vi "array_to_table.vi"() -> ()   [LabVIEW 2022 SP3]
panel:
  out "Table":string[][](table)
  in  "?":dbl[][](array[numeric])
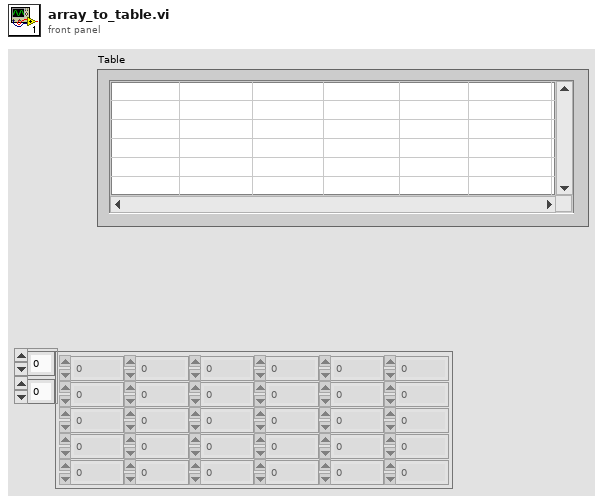
[diagram p1: front panel]
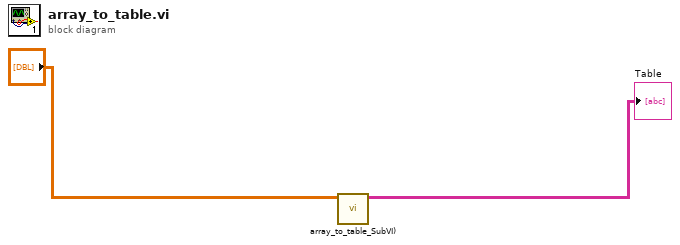
[diagram p0: block diagram]
diagram:
  n1 = call "array_to_table_SubVI).vi"("Array in"="?") -> ("Array out"=→"Table":string[][])  [unwired: 10 in]
